vi "DB Write Queries.vi"(5 "Query info":T1, 7 "COMMAND":T2=enum."TBCALPROC_MCT_TEMP Insert", 8 "에러 입력(에러 없음)":errorcluster, 10 "DATA IN":string[](array[string]), 11 "참조 번호 입력":T3) -> (0 "에러 출력":errorcluster, 3 "참조 번호 출력":T3)   [LabVIEW 2020]
uses:
  <vilib>/addons/database/Connection.llb/Conn ObjectReference.ctl
  Controls/Cmd_Write Query.ctl
  Controls/Clst_Query Info.ctl
  <vilib>/addons/database/Connection.llb/Conn Execute.vi
  <vilib>/addons/database/Recordset.llb/Rec Destroy - Connection.vi
  <vilib>/addons/database/NI_Database_API.lvlib
panel:
  out "Query":string
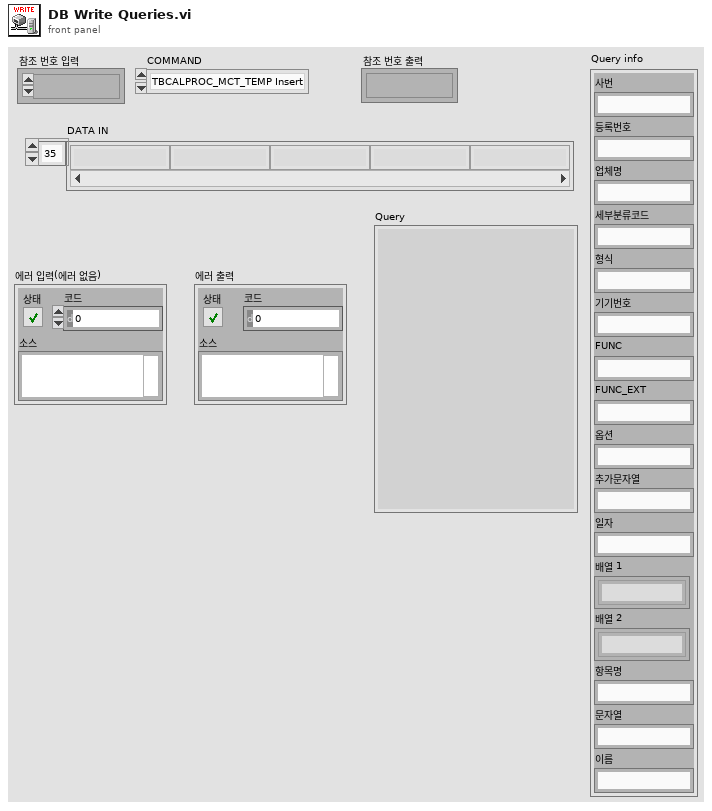
[diagram p1: front panel]
types:
  T1 = typedef "Clst_Query Info.ctl" = cluster{"사번":string, "등록번호":string, "업체명":string, "세부분류코드":string, "형식":string, "기기번호":string, "FUNC":string, "FUNC_EXT":string, "옵션":string, "추가문자열":string, "일자":string, "배열 1":string[], "배열 2":string[], "항목명":string, "문자열":string, "이름":string}
  T2 = typedef "Cmd_Write Query.ctl" = enum16{"TBUSESTD_MCT Insert", "TBUSESTD_MCT Delete", "TBCALSTD_MCT_TEMP Insert", "TBCALSTD_MCT_TEMP Delete", "TBCALSTD_MCT Insert", "TBCALSTD_MCT Delete", "TBCALSTD_MCT_BACK Insert", "TBCALSTD_MCT_BACK Delete", "TBCALPROC_MCT Insert", "TBCALPROC_MCT Delete", "TBCALPROC_MCT_TEMP Insert", "TBCALPROC_MCT_TEMP Delete", "TBCALCMC_MCT Insert", "TBCALCMC_MCT Delete", "TBCALFUNC_MCT Insert", "TBCALFUNC_MCT Delete", "TBCALNAME_MCT Insert", "TBCALNAME_MCT Delete", "TBSTDNAME_MCT Insert", "TBSTDNAME_MCT Delete", "TBCALSPEC_MCT Insert", "TBCALSPEC_MCT Delete", "TBCALSTD_MCT NOTUSE update", "TBCALSPEC_MCT update", "TBMCTVERMAN update"}
  T3 = typedef "NI_Database_API.lvlib/Conn ObjectReference.ctl" = refnum<k1>
  T4 = typedef "NI_Database_API.lvlib/Rec ObjectReference.ctl" = refnum<k1>
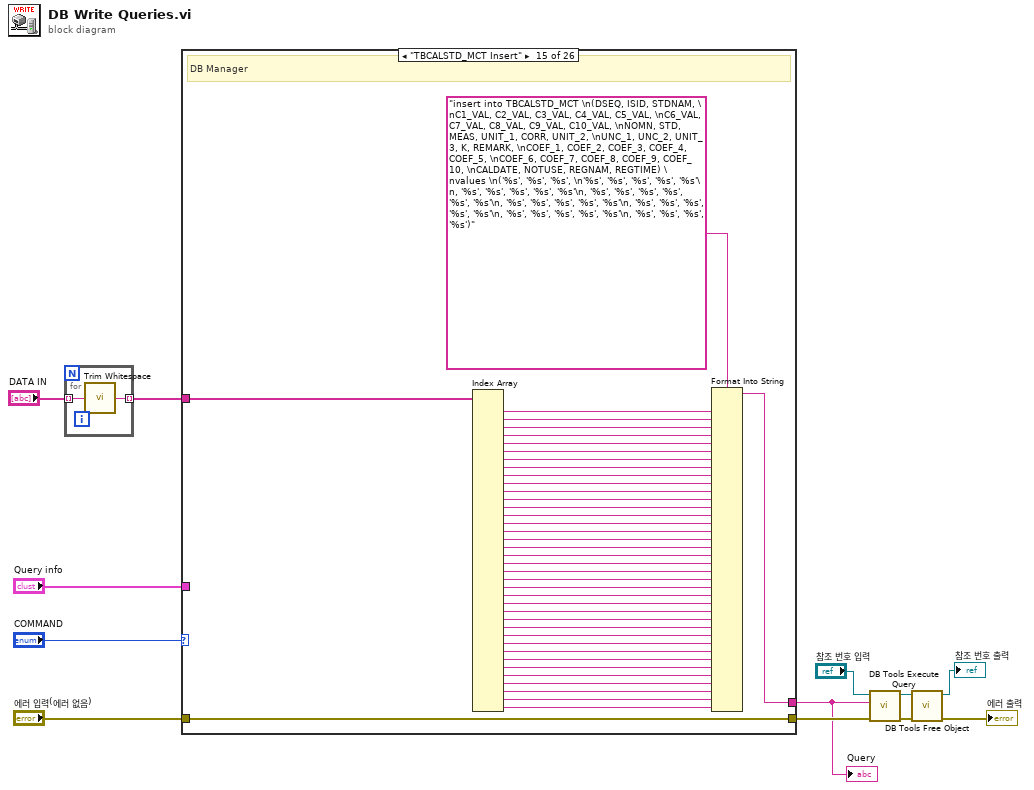
[diagram p0: block diagram]
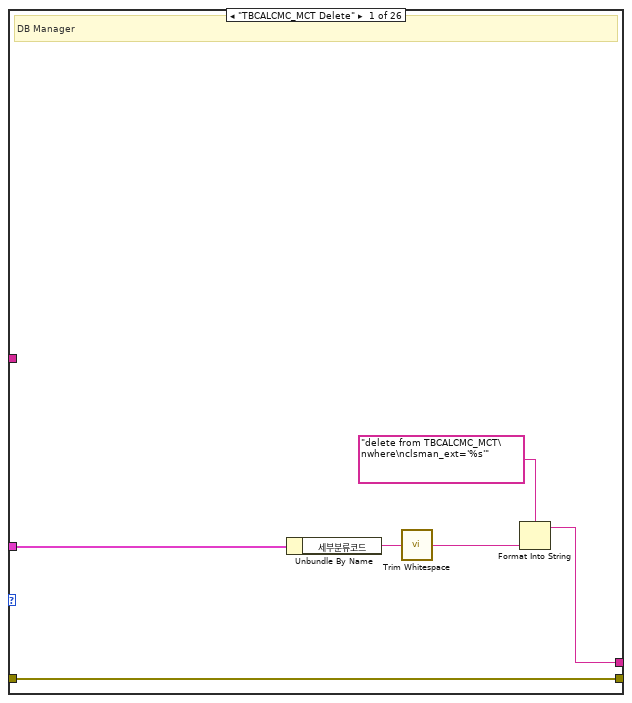
[diagram p2: hidden frame]
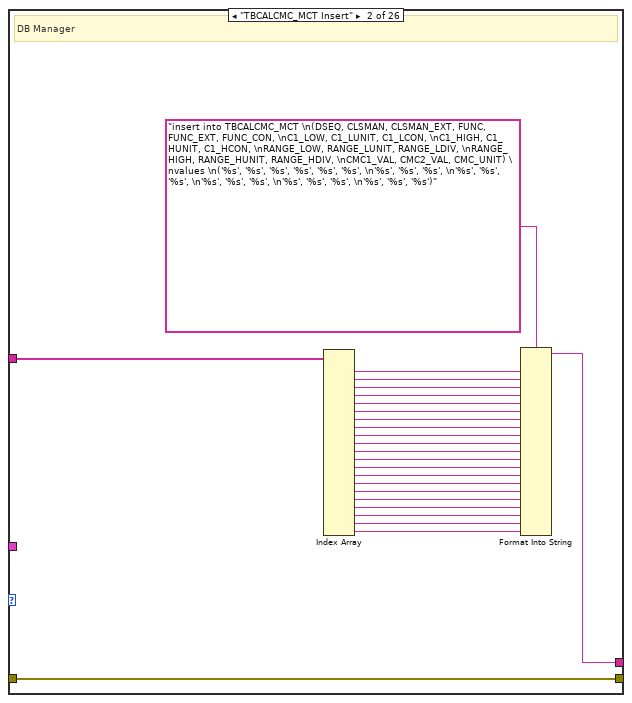
[diagram p3: hidden frame]
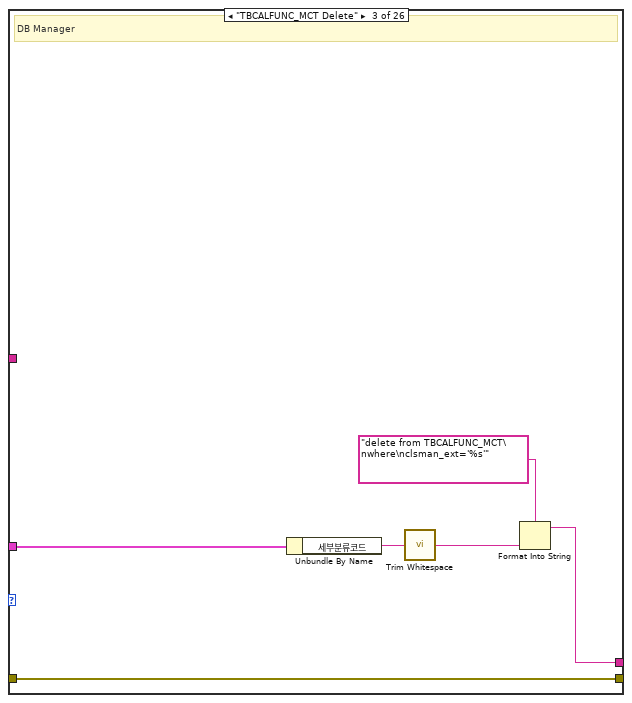
[diagram p4: hidden frame]
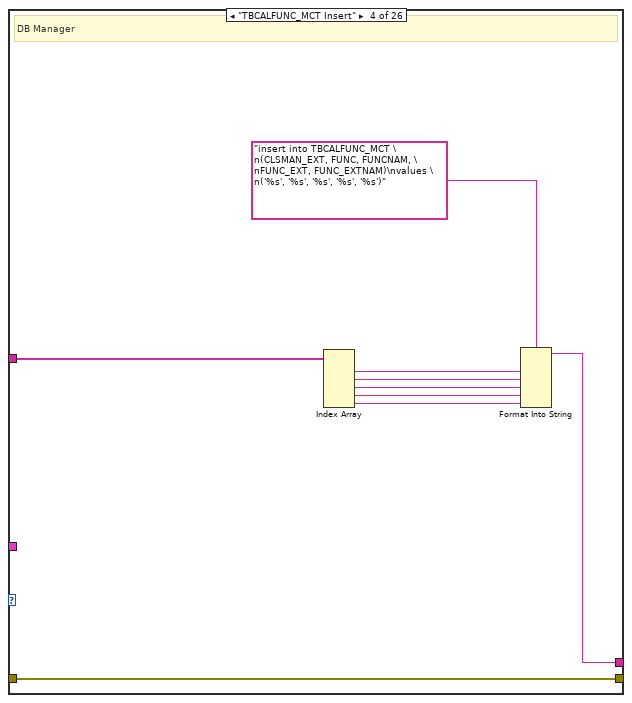
[diagram p5: hidden frame]
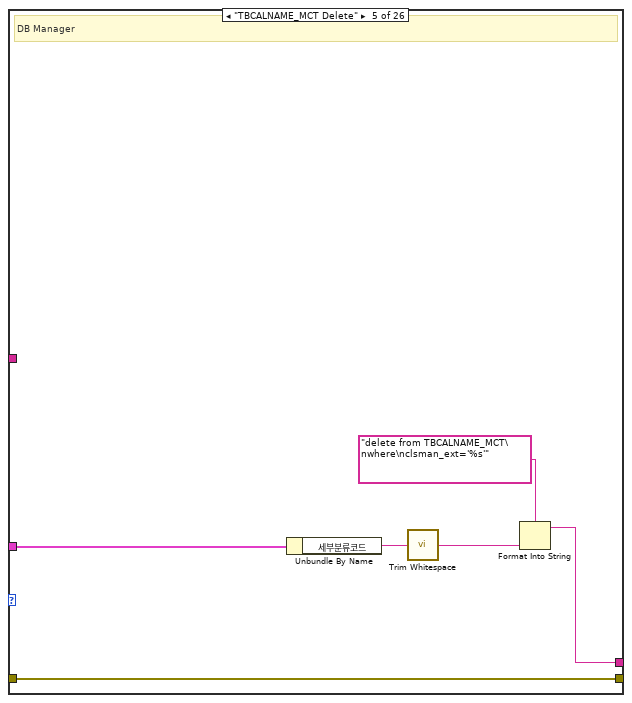
[diagram p6: hidden frame]
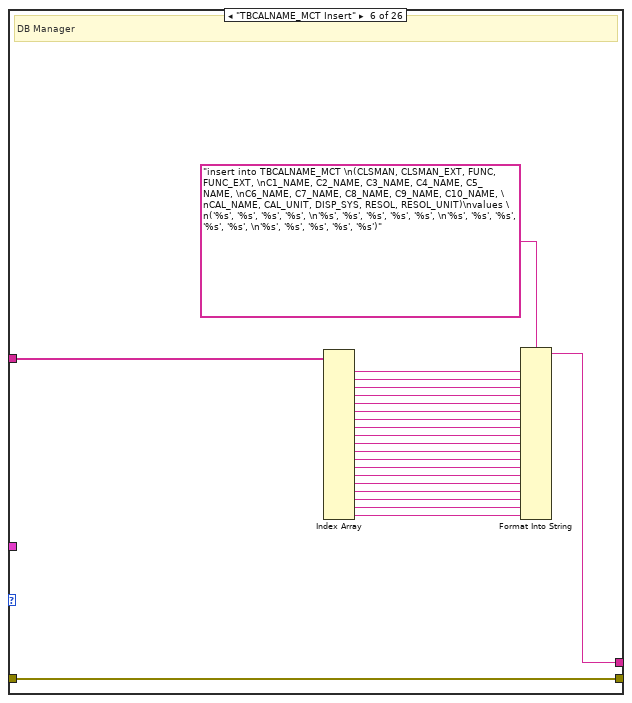
[diagram p7: hidden frame]
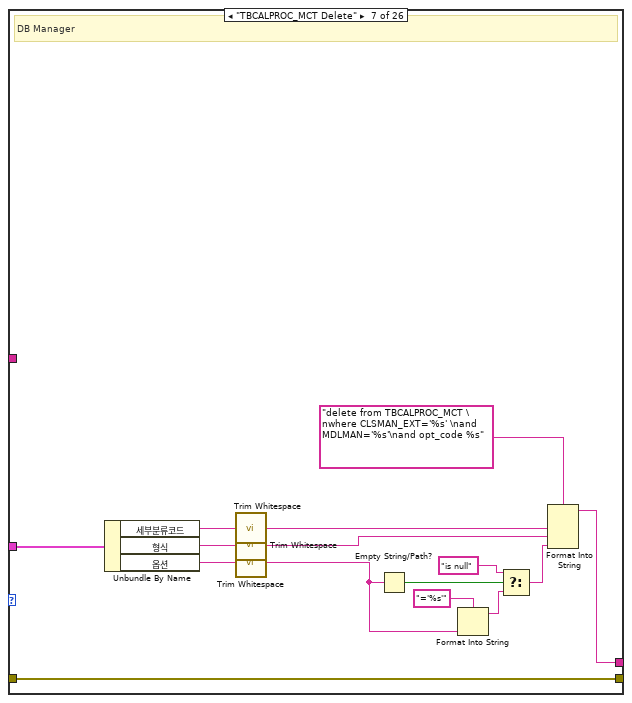
[diagram p8: hidden frame]
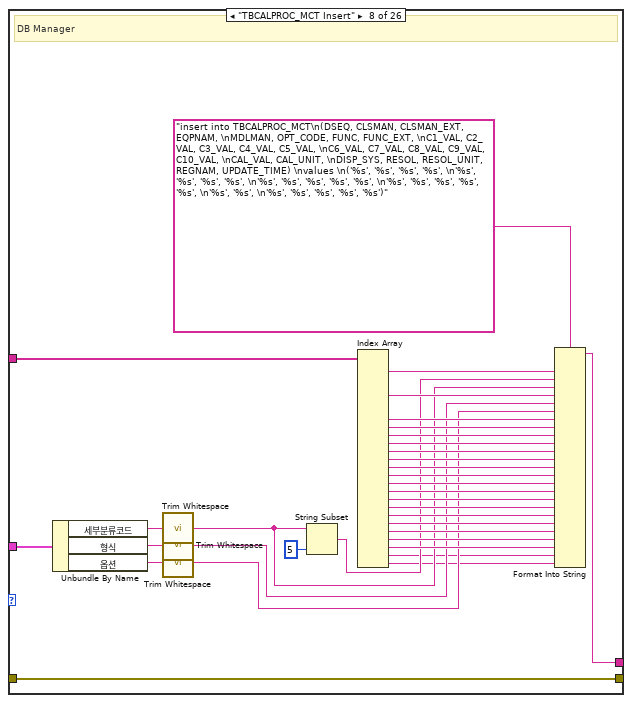
[diagram p9: hidden frame]
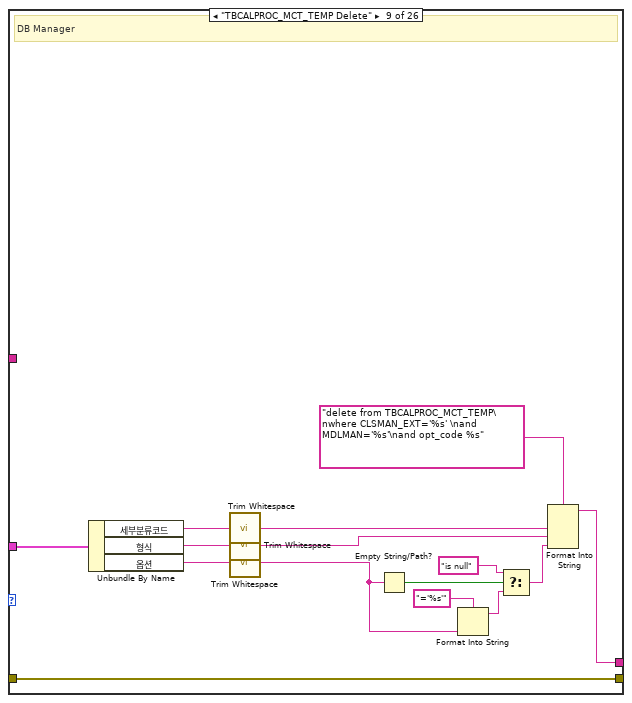
[diagram p10: hidden frame]
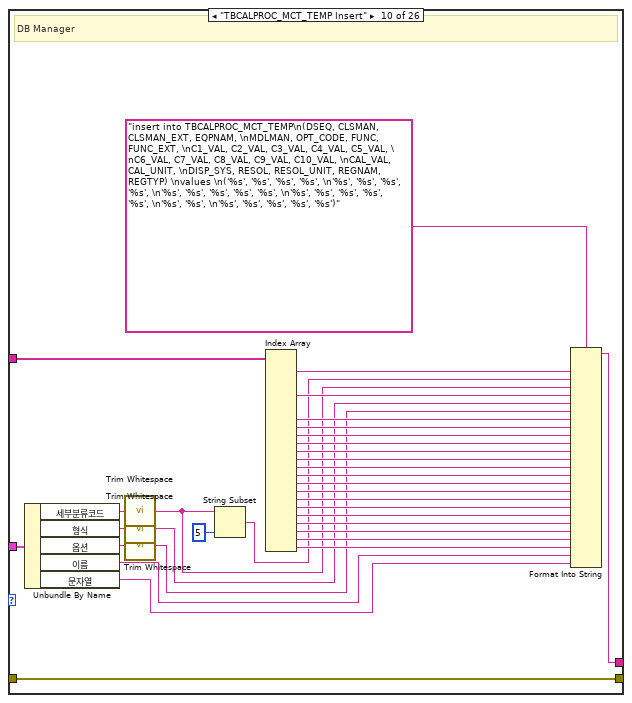
[diagram p11: hidden frame]
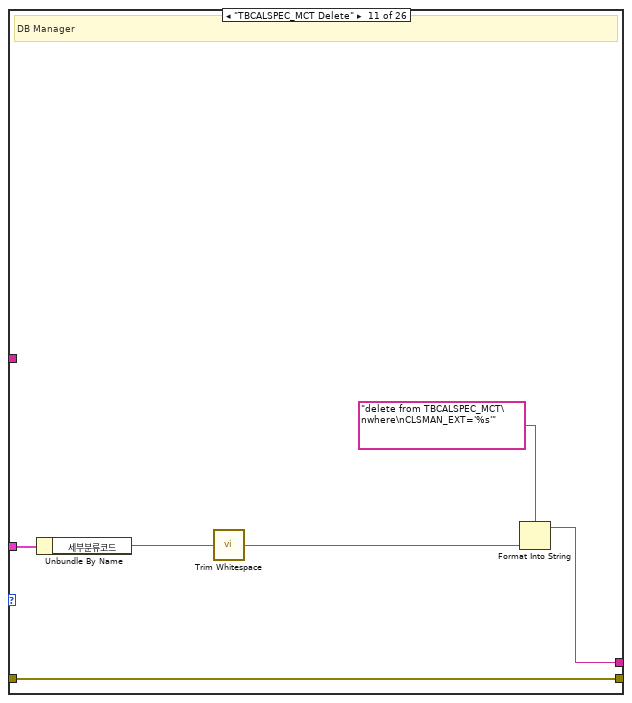
[diagram p12: hidden frame]
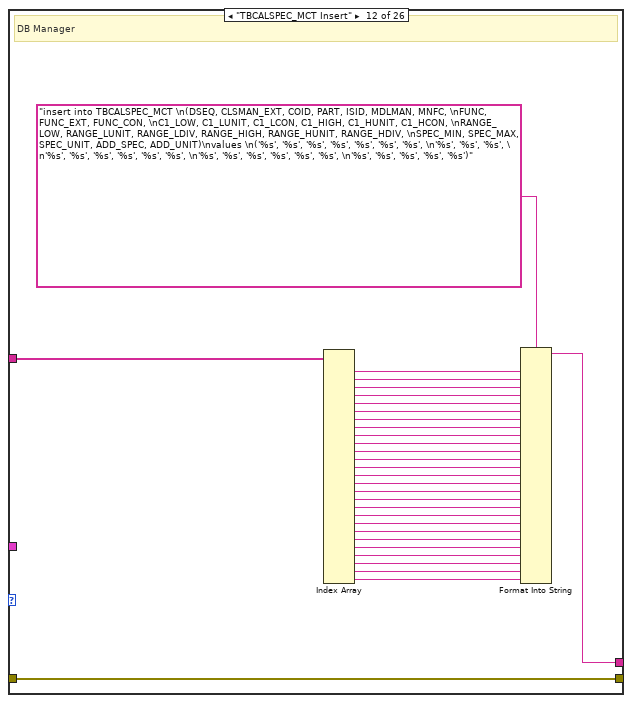
[diagram p13: hidden frame]
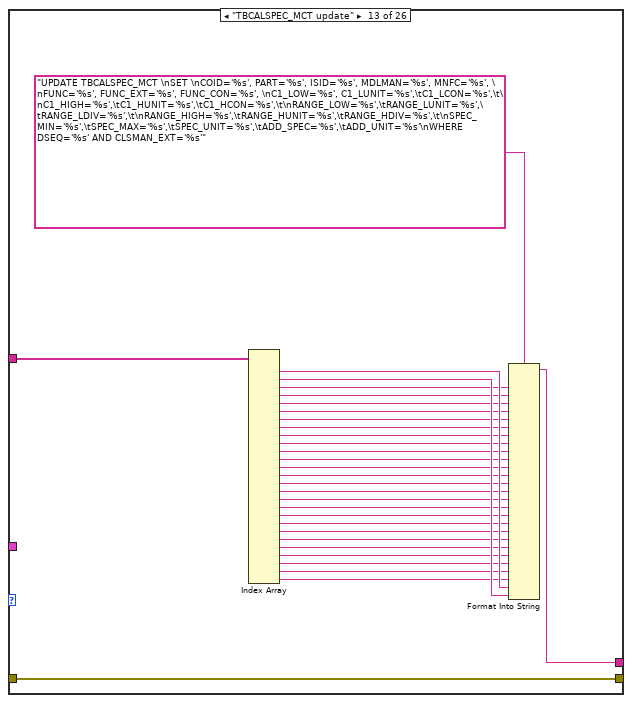
[diagram p14: hidden frame]
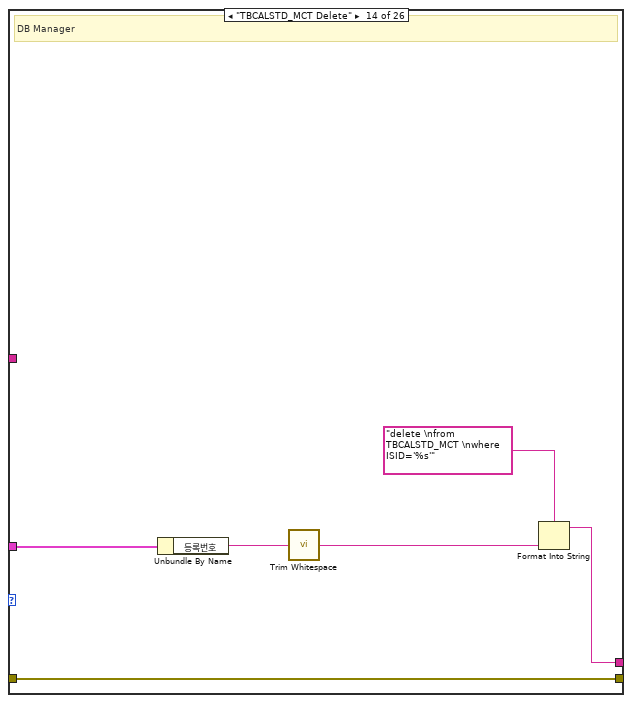
[diagram p15: hidden frame]
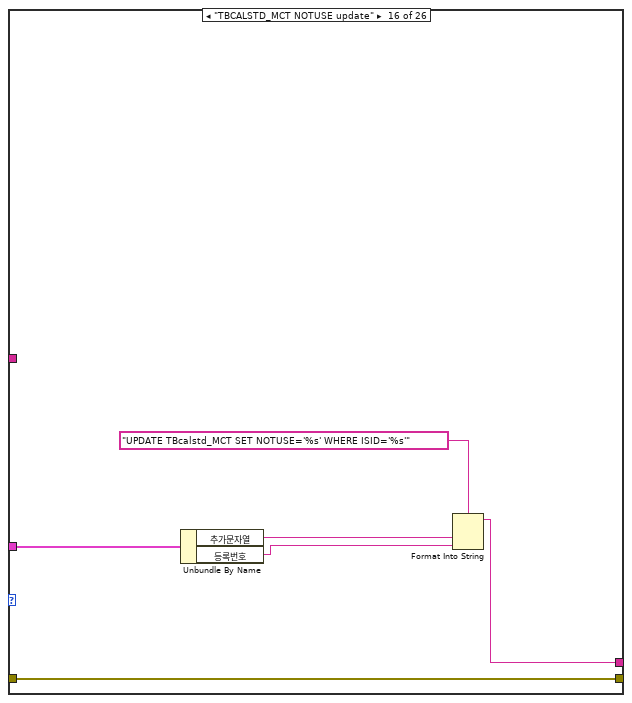
[diagram p16: hidden frame]
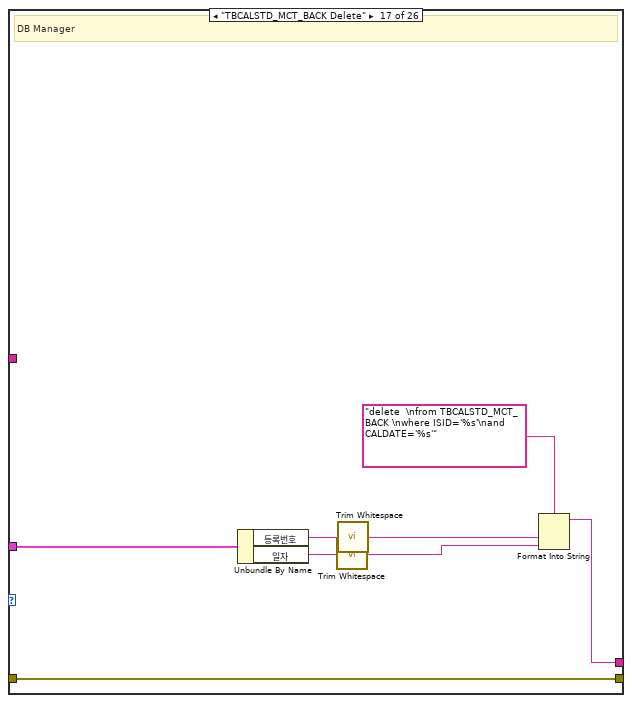
[diagram p17: hidden frame]
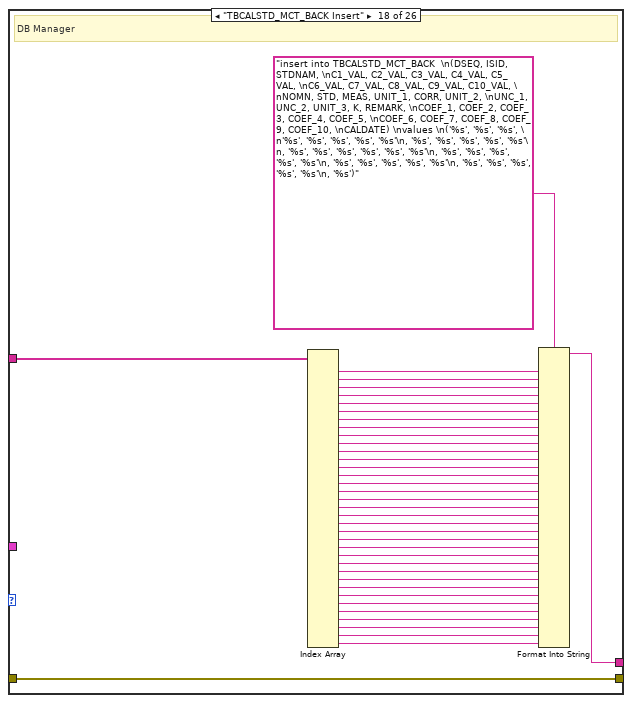
[diagram p18: hidden frame]
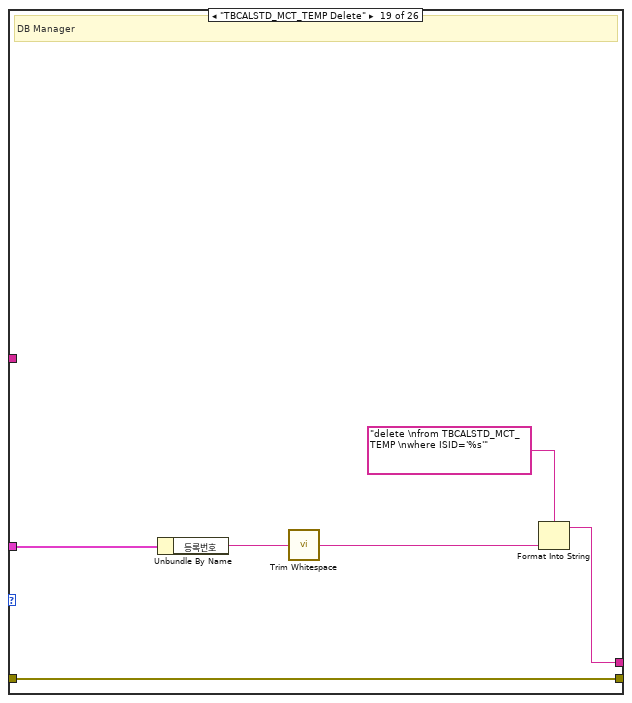
[diagram p19: hidden frame]
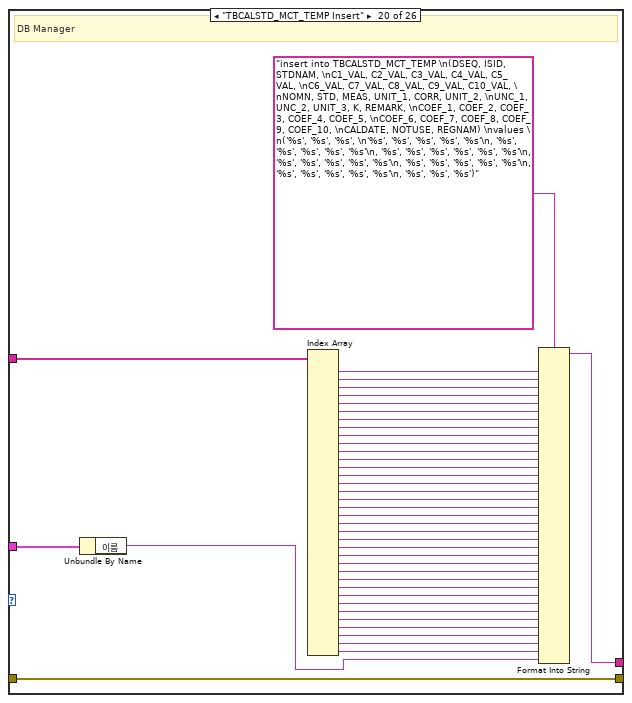
[diagram p20: hidden frame]
diagram:
  n1 = for {
    tunnel: "DATA IN" -> [w14] mode=indexing
    tunnel: [w13] -> w2 mode=indexing
    n2 = call <vilib>:"Trim Whitespace.vi"("string"=w14) -> ("trimmed string"=w13:string)  [unwired: 1 in]
  }
  n3 = case shown="\"TBCALSTD_MCT Insert\"" "COMMAND" {
    tunnel: "에러 입력(에러 없음)" -> [w20 w45 w51 w60 w66 w89 w104 w138 w153 w187 w193 w224 w255 w261 w303 w309 w317 w356 w362 w404 w410 w448 w457 w468 w474 w476]
    tunnel: [w20 w45 w51 w60 w66 w89 w104 w138 w153 w187 w193 w224 w255 w261 w303 w309 w317 w356 w362 w404 w410 w448 w457 w468 w474 w476] -> w7
    tunnel: [w18 w43 w49 w58 w64 w87 w103 w116 w152 w165 w191 w222 w253 w260 w302 w304 w316 w355 w361 w403 w408 w446 w456 w467 w473 "SELECT *\nFROM TBCALCMC_2"] -> w5
    tunnel: w2 -> [_ w42 _ w57 _ w86 _ w117 _ w166 _ w221 w252 _ w300 _ _ w353 _ w401 _ w445 _ w465 _ _]
    tunnel: "Query info" -> [w17 _ w48 _ w63 _ w101 w115 w150 w164 w190 _ _ w258 _ w307 w314 _ w359 w364 w407 _ w454 _ w471 _]
    frame "TBCALCMC_MCT Delete" {
      # "DB Manager"
      n4 = Unbundle By Name(w17) -> ("세부분류코드"=w16:string)
      n5 = call <vilib>:"Trim Whitespace.vi"("string"=w16) -> ("trimmed string"=w15:string)  [unwired: 1 in]
      n6 = Format Into String(format string="delete from TBCALCMC_MCT\nwhere\nclsman_ext='%s'", w15) -> (resulting string=w18:string)  [unwired: 2 in, 1 out]
    }
    frame "TBCALCMC_MCT Insert" {
      # "DB Manager"
      n7 = Index Array(array=w42) -> (element #1=w41:string, element #2=w40:string, element #3=w39:string, element #4=w38:string, element #5=w37:string, element #6=w36:string, element #7=w35:string, element #8=w34:string, element #9=w33:string, element #10=w32:string, element #11=w31:string, element #12=w30:string, element #13=w28:string, element #14=w29:string, element #15=w27:string, element #16=w26:string, element #17=w25:string, element #18=w24:string, element #19=w23:string, element #20=w22:string, element #21=w21:string)  [unwired: 21 in]
      n8 = Format Into String(format string="insert into TBCALCMC_MCT \n(DSEQ, CLSMAN, CLSMAN_EXT, FUNC, FUNC_EXT, FUNC_CON, \nC1_LOW, C1_LUNIT, C1_LCON, \nC1_HIGH, C1_HUNIT, C1_HCON, \nRANGE_LOW, RANGE_LUNIT, RANGE_LDIV, \nRANGE_HIGH, RANGE_HUNIT, RANGE_HDIV, \nCMC1_VAL, CMC2_VAL, CMC_UNIT) \nvalues \n('%s', '%s', '%s', '%s', '%s', '%s', \n'%s', '%s', '%s', \n'%s', '%s', '%s', \n'%s', '%s', '%s', \n'%s', '%s', '%s', \n'%s', '%s', '%s')", w41, w40, w39, w38, w37, w36, w35, w34, w33, w32, w31, w30, w28, w29, w27, w26, w25, w24, w23, w22, w21) -> (resulting string=w43:string)  [unwired: 2 in, 1 out]
    }
    frame "TBCALFUNC_MCT Delete" {
      # "DB Manager"
      n9 = Unbundle By Name(w48) -> ("세부분류코드"=w47:string)
      n10 = call <vilib>:"Trim Whitespace.vi"("string"=w47) -> ("trimmed string"=w46:string)  [unwired: 1 in]
      n11 = Format Into String(format string="delete from TBCALFUNC_MCT\nwhere\nclsman_ext='%s'", w46) -> (resulting string=w49:string)  [unwired: 2 in, 1 out]
    }
    frame "TBCALFUNC_MCT Insert" {
      # "DB Manager"
      n12 = Index Array(array=w57) -> (element #1=w56:string, element #2=w55:string, element #3=w54:string, element #4=w53:string, element #5=w52:string)  [unwired: 5 in]
      n13 = Format Into String(format string="insert into TBCALFUNC_MCT \n(CLSMAN_EXT, FUNC, FUNCNAM, \nFUNC_EXT, FUNC_EXTNAM)\nvalues \n('%s', '%s', '%s', '%s', '%s')", w56, w55, w54, w53, w52) -> (resulting string=w58:string)  [unwired: 2 in, 1 out]
    }
    frame "TBCALNAME_MCT Delete" {
      # "DB Manager"
      n14 = Unbundle By Name(w63) -> ("세부분류코드"=w62:string)
      n15 = call <vilib>:"Trim Whitespace.vi"("string"=w62) -> ("trimmed string"=w61:string)  [unwired: 1 in]
      n16 = Format Into String(format string="delete from TBCALNAME_MCT\nwhere\nclsman_ext='%s'", w61) -> (resulting string=w64:string)  [unwired: 2 in, 1 out]
    }
    frame "TBCALNAME_MCT Insert" {
      # "DB Manager"
      n17 = Index Array(array=w86) -> (element #1=w85:string, element #2=w84:string, element #3=w83:string, element #4=w82:string, element #5=w81:string, element #6=w80:string, element #7=w79:string, element #8=w78:string, element #9=w77:string, element #10=w76:string, element #11=w75:string, element #12=w74:string, element #13=w73:string, element #14=w72:string, element #15=w71:string, element #16=w70:string, element #17=w69:string, element #18=w68:string, element #19=w67:string)  [unwired: 19 in]
      n18 = Format Into String(format string="insert into TBCALNAME_MCT \n(CLSMAN, CLSMAN_EXT, FUNC, FUNC_EXT, \nC1_NAME, C2_NAME, C3_NAME, C4_NAME, C5_NAME, \nC6_NAME, C7_NAME, C8_NAME, C9_NAME, C10_NAME, \nCAL_NAME, CAL_UNIT, DISP_SYS, RESOL, RESOL_UNIT)\nvalues \n('%s', '%s', '%s', '%s', \n'%s', '%s', '%s', '%s', '%s', \n'%s', '%s', '%s', '%s', '%s', \n'%s', '%s', '%s', '%s', '%s')", w85, w84, w83, w82, w81, w80, w79, w78, w77, w76, w75, w74, w73, w72, w71, w70, w69, w68, w67) -> (resulting string=w87:string)  [unwired: 2 in, 1 out]
    }
    frame "TBCALPROC_MCT Delete" {
      # "DB Manager"
      n19 = Unbundle By Name(w101) -> ("세부분류코드"=w100:string, "형식"=w99:string, "옵션"=w94:string)
      n20 = call <vilib>:"Trim Whitespace.vi"("string"=w100) -> ("trimmed string"=w92:string)  [unwired: 1 in]
      n21 = call <vilib>:"Trim Whitespace.vi"("string"=w99) -> ("trimmed string"=w91:string)  [unwired: 1 in]
      n22 = call <vilib>:"Trim Whitespace.vi"("string"=w94) -> ("trimmed string"=w90:string)  [unwired: 1 in]
      n23 = Empty String/Path?(string/path=w90) -> (empty?=w98:bool)
      n24 = Format Into String(format string="='%s'" ("포맷 문자열"), w90) -> (resulting string=w96:string)  [unwired: 2 in, 1 out]
      n25 = Select(t="is null", s=w98, f=w96) -> (s? t:f=w93:string)
      n26 = Format Into String(format string="delete from TBCALPROC_MCT \nwhere CLSMAN_EXT='%s' \nand MDLMAN='%s'\nand opt_code %s", w92, w91, w93) -> (resulting string=w103:string)  [unwired: 2 in, 1 out]
    }
    frame "TBCALPROC_MCT Insert" {
      # "DB Manager"
      n27 = Unbundle By Name(w115) -> ("세부분류코드"=w112:string, "형식"=w114:string, "옵션"=w113:string)
      n28 = call <vilib>:"Trim Whitespace.vi"("string"=w112) -> ("trimmed string"=w109:string)  [unwired: 1 in]
      n29 = call <vilib>:"Trim Whitespace.vi"("string"=w114) -> ("trimmed string"=w108:string)  [unwired: 1 in]
      n30 = call <vilib>:"Trim Whitespace.vi"("string"=w113) -> ("trimmed string"=w107:string)  [unwired: 1 in]
      n31 = String Subset(string=w109, length (rest)=5 ("길이(나머지)")) -> (substring=w110:string)  [unwired: 1 in]
      n32 = Index Array(array=w117) -> (element #1=w136:string, element #4=w135:string, element #7=w134:string, element #8=w133:string, element #9=w132:string, element #10=w131:string, element #11=w130:string, element #12=w129:string, element #13=w127:string, element #14=w128:string, element #15=w126:string, element #16=w125:string, element #17=w124:string, element #18=w123:string, element #19=w122:string, element #20=w121:string, element #21=w120:string, element #22=w119:string, element #23=w118:string, element #24=w105:string, element #25=w106:string)  [unwired: 25 in, 4 out]
      n33 = Format Into String(format string="insert into TBCALPROC_MCT\n(DSEQ, CLSMAN, CLSMAN_EXT, EQPNAM, \nMDLMAN, OPT_CODE, FUNC, FUNC_EXT, \nC1_VAL, C2_VAL, C3_VAL, C4_VAL, C5_VAL, \nC6_VAL, C7_VAL, C8_VAL, C9_VAL, C10_VAL, \nCAL_VAL, CAL_UNIT, \nDISP_SYS, RESOL, RESOL_UNIT, REGNAM, UPDATE_TIME) \nvalues \n('%s', '%s', '%s', '%s', \n'%s', '%s', '%s', '%s', \n'%s', '%s', '%s', '%s', '%s', \n'%s', '%s', '%s', '%s', '%s', \n'%s', '%s', \n'%s', '%s', '%s', '%s', '%s')", w136, w110, w109, w135, w108, w107, w134, w133, w132, w131, w130, w129, w127, w128, w126, w125, w124, w123, w122, w121, w120, w119, w118, w105, w106) -> (resulting string=w116:string)  [unwired: 2 in, 1 out]
    }
    frame "TBCALPROC_MCT_TEMP Delete" {
      # "DB Manager"
      n34 = Unbundle By Name(w150) -> ("세부분류코드"=w149:string, "형식"=w148:string, "옵션"=w143:string)
      n35 = call <vilib>:"Trim Whitespace.vi"("string"=w149) -> ("trimmed string"=w141:string)  [unwired: 1 in]
      n36 = call <vilib>:"Trim Whitespace.vi"("string"=w148) -> ("trimmed string"=w140:string)  [unwired: 1 in]
      n37 = call <vilib>:"Trim Whitespace.vi"("string"=w143) -> ("trimmed string"=w139:string)  [unwired: 1 in]
      n38 = Empty String/Path?(string/path=w139) -> (empty?=w147:bool)
      n39 = Format Into String(format string="='%s'" ("포맷 문자열"), w139) -> (resulting string=w145:string)  [unwired: 2 in, 1 out]
      n40 = Select(t="is null", s=w147, f=w145) -> (s? t:f=w142:string)
      n41 = Format Into String(format string="delete from TBCALPROC_MCT_TEMP\nwhere CLSMAN_EXT='%s' \nand MDLMAN='%s'\nand opt_code %s", w141, w140, w142) -> (resulting string=w152:string)  [unwired: 2 in, 1 out]
    }
    frame "TBCALPROC_MCT_TEMP Insert" {
      # "DB Manager"
      n42 = Unbundle By Name(w164) -> ("세부분류코드"=w161:string, "형식"=w163:string, "옵션"=w162:string, "이름"=w155:string, "문자열"=w154:string)
      n43 = call <vilib>:"Trim Whitespace.vi"("string"=w161) -> ("trimmed string"=w158:string)  [unwired: 1 in]
      n44 = call <vilib>:"Trim Whitespace.vi"("string"=w163) -> ("trimmed string"=w157:string)  [unwired: 1 in]
      n45 = call <vilib>:"Trim Whitespace.vi"("string"=w162) -> ("trimmed string"=w156:string)  [unwired: 1 in]
      n46 = String Subset(string=w158, length (rest)=5 ("길이(나머지)")) -> (substring=w159:string)  [unwired: 1 in]
      n47 = Index Array(array=w166) -> (element #1=w185:string, element #4=w184:string, element #7=w183:string, element #8=w182:string, element #9=w181:string, element #10=w180:string, element #11=w179:string, element #12=w178:string, element #13=w176:string, element #14=w177:string, element #15=w175:string, element #16=w174:string, element #17=w173:string, element #18=w172:string, element #19=w171:string, element #20=w170:string, element #21=w169:string, element #22=w168:string, element #23=w167:string)  [unwired: 23 in, 4 out]
      n48 = Format Into String(format string="insert into TBCALPROC_MCT_TEMP\n(DSEQ, CLSMAN, CLSMAN_EXT, EQPNAM, \nMDLMAN, OPT_CODE, FUNC, FUNC_EXT, \nC1_VAL, C2_VAL, C3_VAL, C4_VAL, C5_VAL, \nC6_VAL, C7_VAL, C8_VAL, C9_VAL, C10_VAL, \nCAL_VAL, CAL_UNIT, \nDISP_SYS, RESOL, RESOL_UNIT, REGNAM, REGTYP) \nvalues \n('%s', '%s', '%s', '%s', \n'%s', '%s', '%s', '%s', \n'%s', '%s', '%s', '%s', '%s', \n'%s', '%s', '%s', '%s', '%s', \n'%s', '%s', \n'%s', '%s', '%s', '%s', '%s')", w185, w159, w158, w184, w157, w156, w183, w182, w181, w180, w179, w178, w176, w177, w175, w174, w173, w172, w171, w170, w169, w168, w167, w155, w154) -> (resulting string=w165:string)  [unwired: 2 in, 1 out]
    }
    frame "TBCALSPEC_MCT Delete" {
      # "DB Manager"
      n49 = Unbundle By Name(w190) -> ("세부분류코드"=w189:string)
      n50 = call <vilib>:"Trim Whitespace.vi"("string"=w189) -> ("trimmed string"=w188:string)  [unwired: 1 in]
      n51 = Format Into String(format string="delete from TBCALSPEC_MCT\nwhere\nCLSMAN_EXT='%s'", w188) -> (resulting string=w191:string)  [unwired: 2 in, 1 out]
    }
    frame "TBCALSPEC_MCT Insert" {
      # "DB Manager"
      n52 = Index Array(array=w221) -> (element #1=w220:string, element #2=w219:string, element #3=w218:string, element #4=w217:string, element #5=w216:string, element #6=w215:string, element #7=w214:string, element #8=w213:string, element #9=w212:string, element #10=w211:string, element #11=w210:string, element #12=w209:string, element #13=w208:string, element #14=w207:string, element #15=w206:string, element #16=w205:string, element #17=w204:string, element #18=w203:string, element #19=w202:string, element #20=w201:string, element #21=w200:string, element #22=w199:string, element #23=w198:string, element #24=w197:string, element #25=w196:string, element #26=w195:string, element #27=w194:string)  [unwired: 27 in]
      n53 = Format Into String(format string="insert into TBCALSPEC_MCT \n(DSEQ, CLSMAN_EXT, COID, PART, ISID, MDLMAN, MNFC, \nFUNC, FUNC_EXT, FUNC_CON, \nC1_LOW, C1_LUNIT, C1_LCON, C1_HIGH, C1_HUNIT, C1_HCON, \nRANGE_LOW, RANGE_LUNIT, RANGE_LDIV, RANGE_HIGH, RANGE_HUNIT, RANGE_HDIV, \nSPEC_MIN, SPEC_MAX, SPEC_UNIT, ADD_SPEC, ADD_UNIT)\nvalues \n('%s', '%s', '%s', '%s', '%s', '%s', '%s', \n'%s', '%s', '%s', \n'%s', '%s', '%s', '%s', '%s', '%s', \n'%s', '%s', '%s', '%s', '%s', '%s', \n'%s', '%s', '%s', '%s', '%s')", w220, w219, w218, w217, w216, w215, w214, w213, w212, w211, w210, w209, w208, w207, w206, w205, w204, w203, w202, w201, w200, w199, w198, w197, w196, w195, w194) -> (resulting string=w222:string)  [unwired: 2 in, 1 out]
    }
    frame "TBCALSPEC_MCT update" {
      n54 = Index Array(array=w252) -> (element #1=w251:string, element #2=w250:string, element #3=w249:string, element #4=w248:string, element #5=w247:string, element #6=w246:string, element #7=w245:string, element #8=w244:string, element #9=w243:string, element #10=w242:string, element #11=w241:string, element #12=w240:string, element #13=w239:string, element #14=w238:string, element #15=w237:string, element #16=w236:string, element #17=w235:string, element #18=w234:string, element #19=w233:string, element #20=w232:string, element #21=w231:string, element #22=w230:string, element #23=w229:string, element #24=w228:string, element #25=w227:string, element #26=w226:string, element #27=w225:string)  [unwired: 27 in]
      n55 = Format Into String(format string="UPDATE TBCALSPEC_MCT \nSET \nCOID='%s', PART='%s', ISID='%s', MDLMAN='%s', MNFC='%s', \nFUNC='%s', FUNC_EXT='%s', FUNC_CON='%s', \nC1_LOW='%s', C1_LUNIT='%s',\tC1_LCON='%s',\t\nC1_HIGH='%s',\tC1_HUNIT='%s',\tC1_HCON='%s',\t\nRANGE_LOW='%s',\tRANGE_LUNIT='%s',\tRANGE_LDIV='%s',\t\nRANGE_HIGH='%s',\tRANGE_HUNIT='%s',\tRANGE_HDIV='%s',\t\nSPEC_MIN='%s',\tSPEC_MAX='%s',\tSPEC_UNIT='%s',\tADD_SPEC='%s',\tADD_UNIT='%s'\nWHERE DSEQ='%s' AND CLSMAN_EXT='%s'" ("포맷 문자열"), w249, w248, w247, w246, w245, w244, w243, w242, w241, w240, w239, w238, w237, w236, w235, w234, w233, w232, w231, w230, w229, w228, w227, w226, w225, w251, w250) -> (resulting string=w253:string)  [unwired: 2 in, 1 out]
    }
    frame "TBCALSTD_MCT Delete" {
      # "DB Manager"
      n56 = Unbundle By Name(w258) -> ("등록번호"=w257:string)
      n57 = call <vilib>:"Trim Whitespace.vi"("string"=w257) -> ("trimmed string"=w256:string)  [unwired: 1 in]
      n58 = Format Into String(format string="delete \nfrom TBCALSTD_MCT \nwhere ISID='%s'" ("포맷 문자열"), w256) -> (resulting string=w260:string)  [unwired: 2 in, 1 out]
    }
    frame "TBCALSTD_MCT Insert" {
      # "DB Manager"
      n59 = Index Array(array=w300) -> (element #1=w299:string, element #2=w298:string, element #3=w297:string, element #4=w296:string, element #5=w295:string, element #6=w294:string, element #7=w293:string, element #8=w292:string, element #9=w291:string, element #10=w290:string, element #11=w289:string, element #12=w288:string, element #13=w287:string, element #14=w286:string, element #15=w285:string, element #16=w284:string, element #17=w283:string, element #18=w282:string, element #19=w281:string, element #20=w280:string, element #21=w279:string, element #22=w278:string, element #23=w277:string, element #24=w276:string, element #25=w275:string, element #26=w274:string, element #27=w273:string, element #28=w272:string, element #29=w271:string, element #30=w270:string, element #31=w269:string, element #32=w268:string, element #33=w267:string, element #34=w266:string, element #35=w265:string, element #36=w264:string, element #37=w263:string, element #38=w262:string)  [unwired: 38 in]
      n60 = Format Into String(format string="insert into TBCALSTD_MCT \n(DSEQ, ISID, STDNAM, \nC1_VAL, C2_VAL, C3_VAL, C4_VAL, C5_VAL, \nC6_VAL, C7_VAL, C8_VAL, C9_VAL, C10_VAL, \nNOMN, STD, MEAS, UNIT_1, CORR, UNIT_2, \nUNC_1, UNC_2, UNIT_3, K, REMARK, \nCOEF_1, COEF_2, COEF_3, COEF_4, COEF_5, \nCOEF_6, COEF_7, COEF_8, COEF_9, COEF_10, \nCALDATE, NOTUSE, REGNAM, REGTIME) \nvalues \n('%s', '%s', '%s', \n'%s', '%s', '%s', '%s', '%s'\n, '%s', '%s', '%s', '%s', '%s'\n, '%s', '%s', '%s', '%s', '%s', '%s'\n, '%s', '%s', '%s', '%s', '%s'\n, '%s', '%s', '%s', '%s', '%s'\n, '%s', '%s', '%s', '%s', '%s'\n, '%s', '%s', '%s', '%s')" ("포맷 문자열"), w299, w298, w297, w296, w295, w294, w293, w292, w291, w290, w289, w288, w287, w286, w285, w284, w283, w282, w281, w280, w279, w278, w277, w276, w275, w274, w273, w272, w271, w270, w269, w268, w267, w266, w265, w264, w263, w262) -> (resulting string=w302:string)  [unwired: 2 in, 1 out]
    }
    frame "TBCALSTD_MCT NOTUSE update" {
      n61 = Unbundle By Name(w307) -> ("추가문자열"=w306:string, "등록번호"=w305:string)
      n62 = Format Into String(format string="UPDATE TBcalstd_MCT SET NOTUSE='%s' WHERE ISID='%s'" ("포맷 문자열"), w306, w305) -> (resulting string=w304:string)  [unwired: 2 in, 1 out]
    }
    frame "TBCALSTD_MCT_BACK Delete" {
      # "DB Manager"
      n63 = Unbundle By Name(w314) -> ("등록번호"=w313:string, "일자"=w312:string)
      n64 = call <vilib>:"Trim Whitespace.vi"("string"=w312) -> ("trimmed string"=w310:string)  [unwired: 1 in]
      n65 = call <vilib>:"Trim Whitespace.vi"("string"=w313) -> ("trimmed string"=w311:string)  [unwired: 1 in]
      n66 = Format Into String(format string="delete  \nfrom TBCALSTD_MCT_BACK \nwhere ISID='%s'\nand CALDATE='%s'" ("포맷 문자열"), w311, w310) -> (resulting string=w316:string)  [unwired: 2 in, 1 out]
    }
    frame "TBCALSTD_MCT_BACK Insert" {
      # "DB Manager"
      n67 = Index Array(array=w353) -> (element #1=w352:string, element #2=w351:string, element #3=w350:string, element #4=w349:string, element #5=w348:string, element #6=w347:string, element #7=w346:string, element #8=w345:string, element #9=w344:string, element #10=w343:string, element #11=w342:string, element #12=w341:string, element #13=w340:string, element #14=w339:string, element #15=w338:string, element #16=w337:string, element #17=w336:string, element #18=w335:string, element #19=w334:string, element #20=w333:string, element #21=w332:string, element #22=w331:string, element #23=w330:string, element #24=w329:string, element #25=w328:string, element #26=w327:string, element #27=w326:string, element #28=w325:string, element #29=w324:string, element #30=w323:string, element #31=w322:string, element #32=w321:string, element #33=w320:string, element #34=w319:string, element #35=w318:string)  [unwired: 35 in]
      n68 = Format Into String(format string="insert into TBCALSTD_MCT_BACK  \n(DSEQ, ISID, STDNAM, \nC1_VAL, C2_VAL, C3_VAL, C4_VAL, C5_VAL, \nC6_VAL, C7_VAL, C8_VAL, C9_VAL, C10_VAL, \nNOMN, STD, MEAS, UNIT_1, CORR, UNIT_2, \nUNC_1, UNC_2, UNIT_3, K, REMARK, \nCOEF_1, COEF_2, COEF_3, COEF_4, COEF_5, \nCOEF_6, COEF_7, COEF_8, COEF_9, COEF_10, \nCALDATE) \nvalues \n('%s', '%s', '%s', \n'%s', '%s', '%s', '%s', '%s'\n, '%s', '%s', '%s', '%s', '%s'\n, '%s', '%s', '%s', '%s', '%s', '%s'\n, '%s', '%s', '%s', '%s', '%s'\n, '%s', '%s', '%s', '%s', '%s'\n, '%s', '%s', '%s', '%s', '%s'\n, '%s')" ("포맷 문자열"), w352, w351, w350, w349, w348, w347, w346, w345, w344, w343, w342, w341, w340, w339, w338, w337, w336, w335, w334, w333, w332, w331, w330, w329, w328, w327, w326, w325, w324, w323, w322, w321, w320, w319, w318) -> (resulting string=w355:string)  [unwired: 2 in, 1 out]
    }
    frame "TBCALSTD_MCT_TEMP Delete" {
      # "DB Manager"
      n69 = Unbundle By Name(w359) -> ("등록번호"=w358:string)
      n70 = call <vilib>:"Trim Whitespace.vi"("string"=w358) -> ("trimmed string"=w357:string)  [unwired: 1 in]
      n71 = Format Into String(format string="delete \nfrom TBCALSTD_MCT_TEMP \nwhere ISID='%s'" ("포맷 문자열"), w357) -> (resulting string=w361:string)  [unwired: 2 in, 1 out]
    }
    frame "TBCALSTD_MCT_TEMP Insert" {
      # "DB Manager"
      n72 = Unbundle By Name(w364) -> ("이름"=w363:string)
      n73 = Index Array(array=w401) -> (element #1=w400:string, element #2=w399:string, element #3=w398:string, element #4=w397:string, element #5=w396:string, element #6=w395:string, element #7=w394:string, element #8=w393:string, element #9=w392:string, element #10=w391:string, element #11=w390:string, element #12=w389:string, element #13=w388:string, element #14=w387:string, element #15=w386:string, element #16=w385:string, element #17=w384:string, element #18=w383:string, element #19=w382:string, element #20=w381:string, element #21=w380:string, element #22=w379:string, element #23=w378:string, element #24=w377:string, element #25=w376:string, element #26=w375:string, element #27=w374:string, element #28=w373:string, element #29=w372:string, element #30=w371:string, element #31=w370:string, element #32=w369:string, element #33=w368:string, element #34=w367:string, element #35=w366:string, element #36=w365:string)  [unwired: 36 in]
      n74 = Format Into String(format string="insert into TBCALSTD_MCT_TEMP \n(DSEQ, ISID, STDNAM, \nC1_VAL, C2_VAL, C3_VAL, C4_VAL, C5_VAL, \nC6_VAL, C7_VAL, C8_VAL, C9_VAL, C10_VAL, \nNOMN, STD, MEAS, UNIT_1, CORR, UNIT_2, \nUNC_1, UNC_2, UNIT_3, K, REMARK, \nCOEF_1, COEF_2, COEF_3, COEF_4, COEF_5, \nCOEF_6, COEF_7, COEF_8, COEF_9, COEF_10, \nCALDATE, NOTUSE, REGNAM) \nvalues \n('%s', '%s', '%s', \n'%s', '%s', '%s', '%s', '%s'\n, '%s', '%s', '%s', '%s', '%s'\n, '%s', '%s', '%s', '%s', '%s', '%s'\n, '%s', '%s', '%s', '%s', '%s'\n, '%s', '%s', '%s', '%s', '%s'\n, '%s', '%s', '%s', '%s', '%s'\n, '%s', '%s', '%s')" ("포맷 문자열"), w400, w399, w398, w397, w396, w395, w394, w393, w392, w391, w390, w389, w388, w387, w386, w385, w384, w383, w382, w381, w380, w379, w378, w377, w376, w375, w374, w373, w372, w371, w370, w369, w368, w367, w366, w365, w363) -> (resulting string=w403:string)  [unwired: 2 in, 1 out]
    }
    frame "TBSTDNAME_MCT Delete" {
      # "DB Manager"
      n75 = Unbundle By Name(w407) -> ("추가문자열"=w406:string)
      n76 = call <vilib>:"Trim Whitespace.vi"("string"=w406) -> ("trimmed string"=w405:string)  [unwired: 1 in]
      n77 = Format Into String(format string="delete from TBSTDNAME_MCT\nwhere\nSTDNAM='%s'", w405) -> (resulting string=w408:string)  [unwired: 2 in, 1 out]
    }
    frame "TBSTDNAME_MCT Insert" {
      # "DB Manager"
      n78 = Index Array(array=w445) -> (element #1=w444:string, element #2=w443:string, element #3=w442:string, element #4=w441:string, element #5=w440:string, element #6=w439:string, element #7=w438:string, element #8=w437:string, element #9=w436:string, element #10=w435:string, element #11=w434:string, element #12=w433:string, element #13=w432:string, element #14=w431:string, element #15=w430:string, element #16=w429:string, element #17=w428:string, element #18=w427:string, element #19=w426:string, element #20=w425:string, element #21=w424:string, element #22=w423:string, element #23=w422:string, element #24=w421:string, element #25=w420:string, element #26=w419:string, element #27=w418:string, element #28=w417:string, element #29=w416:string, element #30=w415:string, element #31=w414:string, element #32=w413:string, element #33=w412:string, element #34=w411:string)  [unwired: 34 in]
      n79 = Format Into String(format string="insert into TBSTDNAME_MCT \n(STDNAM, C1_VAL, C2_VAL, C3_VAL, C4_VAL, C5_VAL, \nC6_VAL, C7_VAL, C8_VAL, C9_VAL, C10_VAL, \nNOMN, STD, MEAS, UNIT_1, CORR, UNIT_2, \nUNC_1, UNC_2, UNIT_3, K, REMARK, \nCOEF_1, COEF_2, COEF_3, COEF_4, COEF_5, \nCOEF_6, COEF_7, COEF_8, COEF_9, COEF_10, \nCALDATE, NOTUSE)\nvalues \n('%s', '%s', '%s', '%s', '%s', '%s', \n'%s', '%s', '%s', '%s', '%s', \n'%s', '%s', '%s', '%s', '%s', '%s', \n'%s', '%s', '%s', '%s', '%s',\n'%s', '%s', '%s', '%s', '%s', \n'%s', '%s', '%s', '%s', '%s', \n'%s', '%s' )", w444, w443, w442, w441, w440, w439, w438, w437, w436, w435, w434, w433, w432, w431, w430, w429, w428, w427, w426, w425, w424, w423, w422, w421, w420, w419, w418, w417, w416, w415, w414, w413, w412, w411) -> (resulting string=w446:string)  [unwired: 2 in, 1 out]
    }
    frame "TBUSESTD_MCT Delete" {
      # "DB Manager"
      n80 = Unbundle By Name(w454) -> ("세부분류코드"=w453:string, "FUNC"=w451:string)
      n81 = call <vilib>:"Trim Whitespace.vi"("string"=w451) -> ("trimmed string"=w450:string)  [unwired: 1 in]
      n82 = call <vilib>:"Trim Whitespace.vi"("string"=w453) -> ("trimmed string"=w452:string)  [unwired: 1 in]
      n83 = case shown="기본" w450 {
        selector: w450 -> [w460 _]
        tunnel: [w459 _] -> w449
        frame Default {
          n84 = Format Into String(format string="and FUNC='%s'" ("포맷 문자열"), w460) -> (resulting string=w459:string)  [unwired: 2 in, 1 out]
        }
        frame "" {
        }
      }
      n85 = Format Into String(format string="delete \nfrom TBUSESTD_MCT \nwhere CLSMAN_EXT='%s'\n%s" ("포맷 문자열"), w452, w449) -> (resulting string=w456:string)  [unwired: 2 in, 1 out]
    }
    frame "TBUSESTD_MCT Insert" {
      # "DB Manager"
      n86 = Index Array(array=w465) -> (element #1=w461:string, element #2=w464:string, element #4=w462:string, element #6=w463:string)  [unwired: 6 in, 2 out]
      n87 = Format Into String(format string="insert into TBUSESTD_MCT \n(CLSMAN_EXT, FUNC, FUNC_EXT, STDNAM) \nvalues \n('%s', '%s', '%s', '%s')" ("포맷 문자열"), w461, w464, w462, w463) -> (resulting string=w467:string)  [unwired: 2 in, 1 out]
    }
    frame "TBMCTVERMAN update" {
      # "DB Manager"
      n88 = Unbundle By Name(w471) -> ("추가문자열"=w469:string, "문자열"=w470:string)
      n89 = Format Into String(format string="UPDATE TBMCTVERMAN SET %s_VER='%s'" ("포맷 문자열"), w469, w470) -> (resulting string=w473:string)  [unwired: 2 in, 1 out]
    }
    frame Default {
    }
  }
  "Query" <- w5
  n90 = call-poly <vilib>:"DB Tools Execute Query.vi"("error in (no error)"=w7, "SQL query"=w5, "connection reference"="참조 번호 입력") -> ("error out"=w6:errorcluster, "recordset reference"=w9:T4)  [unwired: 5 in]
  n91 = call-poly <vilib>:"DB Tools Free Object.vi"("error in (no error)"=w6, "recordset reference"=w9) -> ("error out"=→"에러 출력":errorcluster, "connection reference"=→"참조 번호 출력":T3)  [unwired: 8 in]
